vi "Actor Core.vi"(8 "error in":errorcluster, 11 "TestBench in":refnum<class "TestBench.lvclass">) -> (0 "error out":errorcluster, 3 "Actor out":refnum<class "Actor.lvclass">)   [LabVIEW 2019, in "TestBench.lvlib" / "TestBench.lvclass"]
doc: "(<B>Filename</B>: Actor Framework.lvlib:Actor.lvclass:Actor Core.vi)\n\nReceives messages to the actor, reacts to them, and initiates any error handling that may shut the actor down.\n\nDescendant classes may override this VI to append parallel tasks for the actor to complete while it handles messages. Overrides use the Call Parent Method node."
uses:
  TestBench.lvclass
  C:/Program Files (x86)/National Instruments/LabVIEW 2019/vi.lib/ActorFramework/Actor/Actor.lvclass
  <vilib>/ActorFramework/Actor/Actor.lvclass
  DataBase/DataBase/DataBase.lvclass
  EventRecorder/EventRecorder/EventRecorder.lvclass
  TestSetup/TestSetup/TestSetup.lvclass
  UserManagement/UserManagement/UserManagement.lvclass
  LocalReport/LocalReport/LocalReport.lvclass
  SignalProcessing/SignalProcessing/SignalProcessing.lvclass
  SoftwareSetup/SoftwareSetup/SoftwareSetup.lvclass
  SoftwareSetup/SoftwareSetup/DataBase.ctl
  SoftwareSetup/SoftwareSetup/Local Report.ctl
  SoftwareSetup/SoftwareSetup/Localization.ctl
  SoftwareSetup/SoftwareSetup/Preferences.ctl
  SoftwareSetup/SoftwareSetup/User Manager.ctl
  SoftwareSetup/SoftwareSetup/Multiple UUT Settings.ctl
  SoftwareSetup/SoftwareSetup/Sequence.ctl
  SystemSetup/SystemSetup/SystemSetup.lvclass
  Assert/Assert/Assert.lvclass
  TestRunner/TestRunner/TestRunner.lvclass
  TestBench.lvclass/TestBench.ctl
  HardwareSetup_model001/HardwareSetup_modle001/HardwareSetup_model001.lvclass
  D:/TestBench/SystemSetup/SystemSetup/SystemSetup.lvclass
  <vilib>/ActorFramework/Actor/Actor.lvclass/Actor.ctl
  <vilib>/ActorFramework/Message Enqueuer/Message Enqueuer.lvclass/Message Enqueuer.ctl
  UserManagement/UserManagement Messages/ActorCoreMassageEvent Msg/ActorCoreMassageEvent Msg.lvclass/ActorCoreMassageEvent Msg.ctl
  SystemSetup/SystemSetup Messages/ActorCoreEvent Msg/ActorCoreEvent Msg.lvclass/ActorCoreEvent Msg.ctl
  EventRecorder/EventRecorder Messages/ActorCoreEvent Msg/ActorCoreEvent Msg.lvclass/ActorCoreEvent Msg.ctl
  DataBase/DataBase Messages/ActorCoreEvent Msg/ActorCoreEvent Msg.lvclass/ActorCoreEvent Msg.ctl
  LocalReport/LocalReport Messages/InitializeReport Msg/InitializeReport Msg.lvclass/InitializeReport Msg.ctl
  DataBase/DataBase Messages/Initialize Msg/Initialize Msg.lvclass/Initialize Msg.ctl
  89e34157-fbcc-4783-a5bd-c972c4c63c1c.vi
  <vilib>/ActorFramework/Message Enqueuer/Init from Existing Queue.vi
  <vilib>/ActorFramework/Message Enqueuer/Enqueue.vi
  TestBench Messages/Stop Test Engine Actor Msg/Stop Test Engine Actor Msg.lvclass
  C:/Program Files (x86)/National Instruments/LabVIEW 2019/vi.lib/ActorFramework/Message/Message.lvclass
  <vilib>/ActorFramework/Stop Msg/Stop Msg.lvclass
  TestBench Messages/UI Initialize Msg/UI Initialize Msg.lvclass
  UserManagement/UserManagement Messages/Login Msg/Login Msg.lvclass
  TestBench Messages/Logout Msg/Logout Msg.lvclass
  UserManagement/UserManagement Messages/ActorCoreMassageEvent Msg/ActorCoreMassageEvent Msg.lvclass
  SystemSetup/SystemSetup Messages/ActorCoreEvent Msg/ActorCoreEvent Msg.lvclass
  EventRecorder/EventRecorder Messages/ActorCoreEvent Msg/ActorCoreEvent Msg.lvclass
  DataBase/DataBase Messages/ActorCoreEvent Msg/ActorCoreEvent Msg.lvclass
  TestBench Messages/Terminate Test Msg/Terminate Test Msg.lvclass
  TestBench Messages/SelectProductModle Msg/SelectProductModel Msg.lvclass
  TestBench Messages/ReadSerialNumber Msg/ReadSerialNumber Msg.lvclass
  LocalReport/LocalReport Messages/InitializeReport Msg/InitializeReport Msg.lvclass
  TestBench Messages/LunchTest Msg/LunchTest Msg.lvclass
  TestBench Messages/Change Sub Panel VI Msg/Change Sub Panel VI Msg.lvclass
  TestBench Messages/PopUp Msg/PopUp Msg.lvclass
  DataBase/DataBase Messages/Initialize Msg/Initialize Msg.lvclass
  <vilib>/ActorFramework/Message Priority Queue/Priority Enqueue.vi
  <vilib>/ActorFramework/Message Enqueuer/Message Enqueuer.lvclass
  SoftwareSetup/SoftwareSetup.lvlib
panel:
  in  "Socket List":i32(listbox)
  in  "Reconnection MySQL":bool
  in  "ShowScannerDialog":bool
  out "Slide":u32(slide)=17 scale=0.0..100.0
  out "CycleTime":dbl format="%.3f(s)"
  in  "Launch":bool
  in  "Break on Failure":enum32{"Yes", "No"}(radio)
  out "ProductType":string
  out "SequencePath":string
  out "Statistics":T1 {"Total" format="Total: %d"; "Yield" format="Yield: %.2f"; "Failed" format="Failed: %d"; "Pass" format="Pass: %d"}
  out "UserName":string
  out "StateBar":string
  # "SequencePath"
  # "ProductType"
  # "CycleTime"
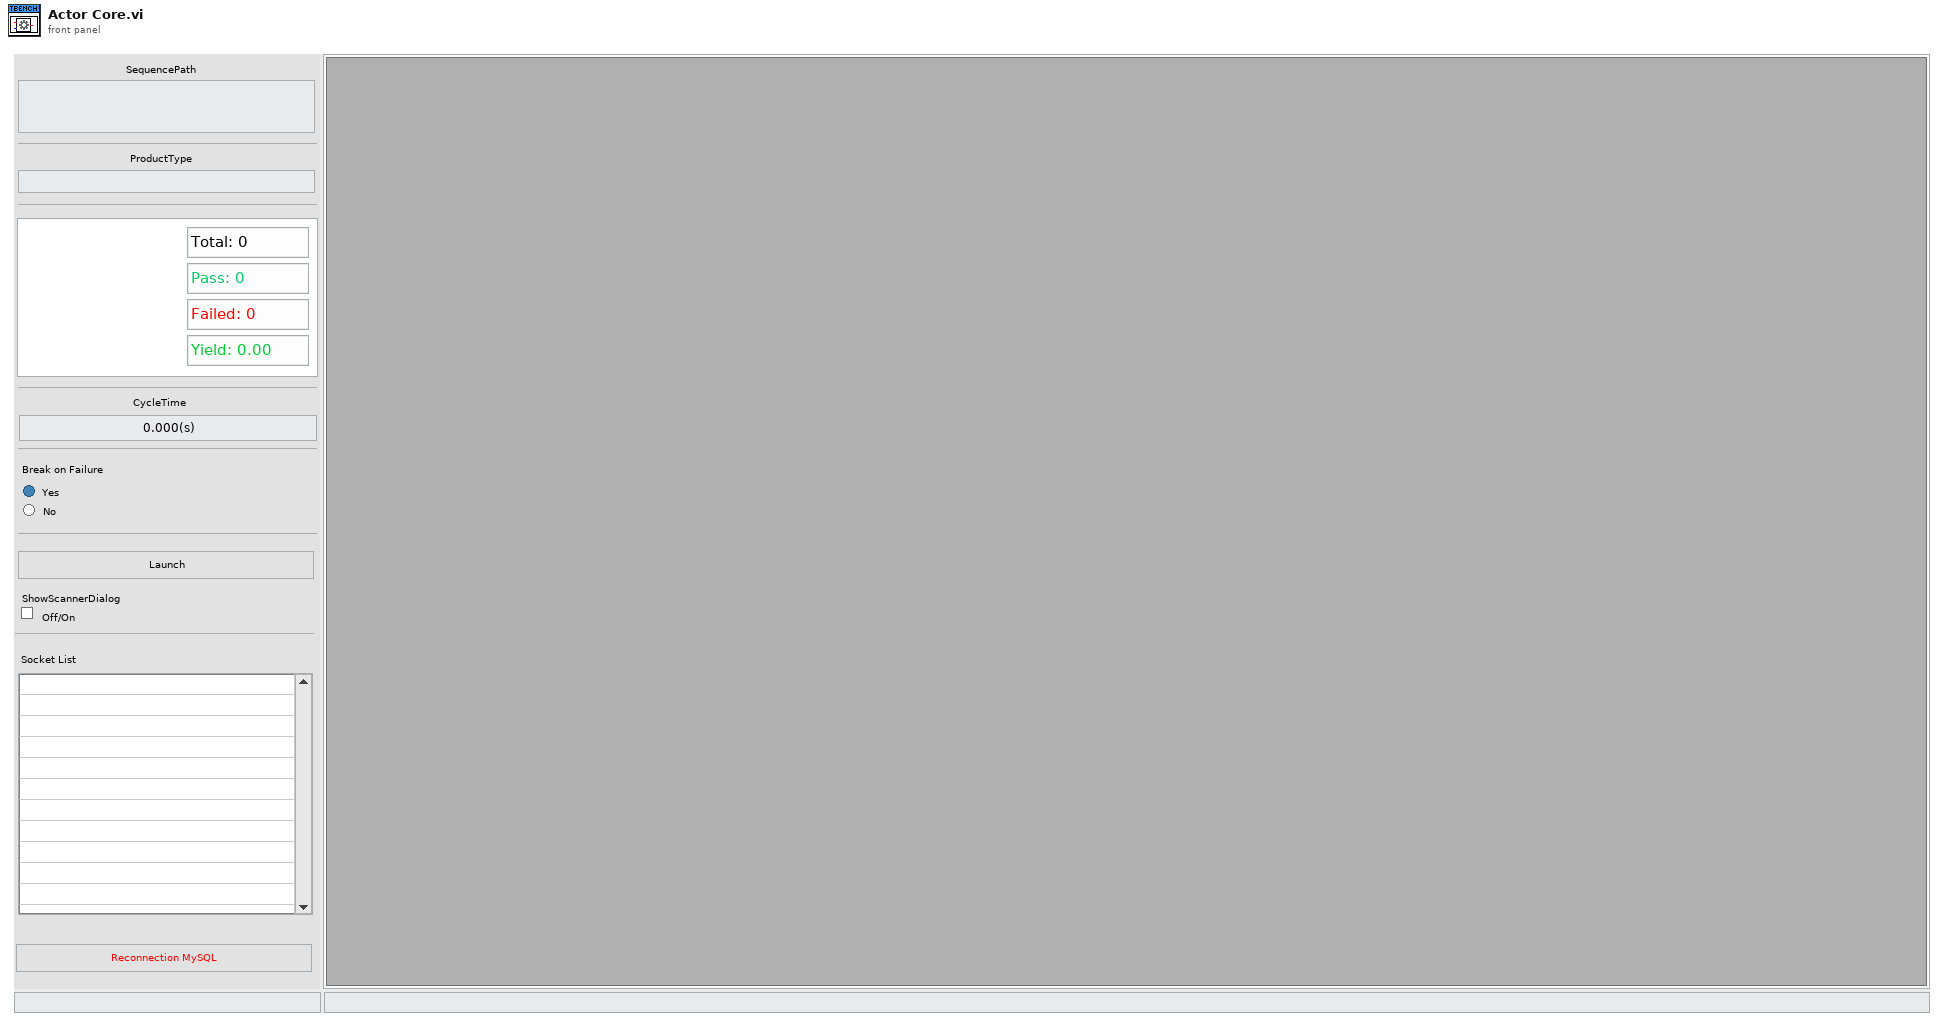
[diagram p1: front panel]
types:
  T1 = cluster{"2D Picture":picture, "Pass":u32, "Failed":u32, "Yield":dbl, "Total":u32}
  T2 = typedef "SoftwareSetup.lvlib/DataBase.ctl" = cluster{"Connection String Expression":string, "User ID":string, "Password":string}
  T3 = typedef "SoftwareSetup.lvlib/Local Report.ctl" = cluster{"Report Path":path, "Report  Format":enum16{"CSV", "XML", "PDF", "Excel", "TXT"}, "Disabled State":bool, "Customer name":string}
  T4 = typedef "SoftwareSetup.lvlib/Localization.ctl" = cluster{"Language":enum16{"English", "Chinese"}}
  T5 = typedef "SoftwareSetup.lvlib/Preferences.ctl" = cluster{"Station ID":string, "IP Address":string, "Password":string}
  T6 = typedef "SoftwareSetup.lvlib/User Manager.ctl" = cluster{"Current User Manager File":string, "Login on start":bool}
  T7 = typedef "SoftwareSetup.lvlib/Multiple UUT Settings.ctl" = cluster{"Number of Tests Sockets":u8, "Synchronization":enum16{"Don't Synchronize", "Serial", "Parallel", "One Thread Only"}}
  T8 = typedef "SoftwareSetup.lvlib/Sequence.ctl" = cluster{"Sequence Folder Path":path}
  T9 = cluster{"DataBase":T2, "Local Report":T3, "Localization":T4, "Preferences":T5, "User Manager":T6, "Multiple UUT Settings":T7, "Sequence":T8}
  T10 = enum32{"Invalid", "Standard", "Closed", "Hidden", "Minimized", "Maximized"}
  T11 = enum32{"invalid app kind", "Development System", "Run Time System", "Student Edition", "Embedded LabVIEW", "Evaluation", "Custom"}
  T12 = cluster{"User ID":string, "ConnectString":string, "Password":string}
  T13 = cluster{"Core":cluster{"Current VI Reference":refnum<vi>, "Close Panel on Exit?":bool}, "DataBase":T2, "Local Report":T3, "Localization":T4, "Preferences":T5, "User Manager":T6}
  T14 = cluster{"Current VI Reference":refnum<vi>, "Close Panel on Exit?":bool}
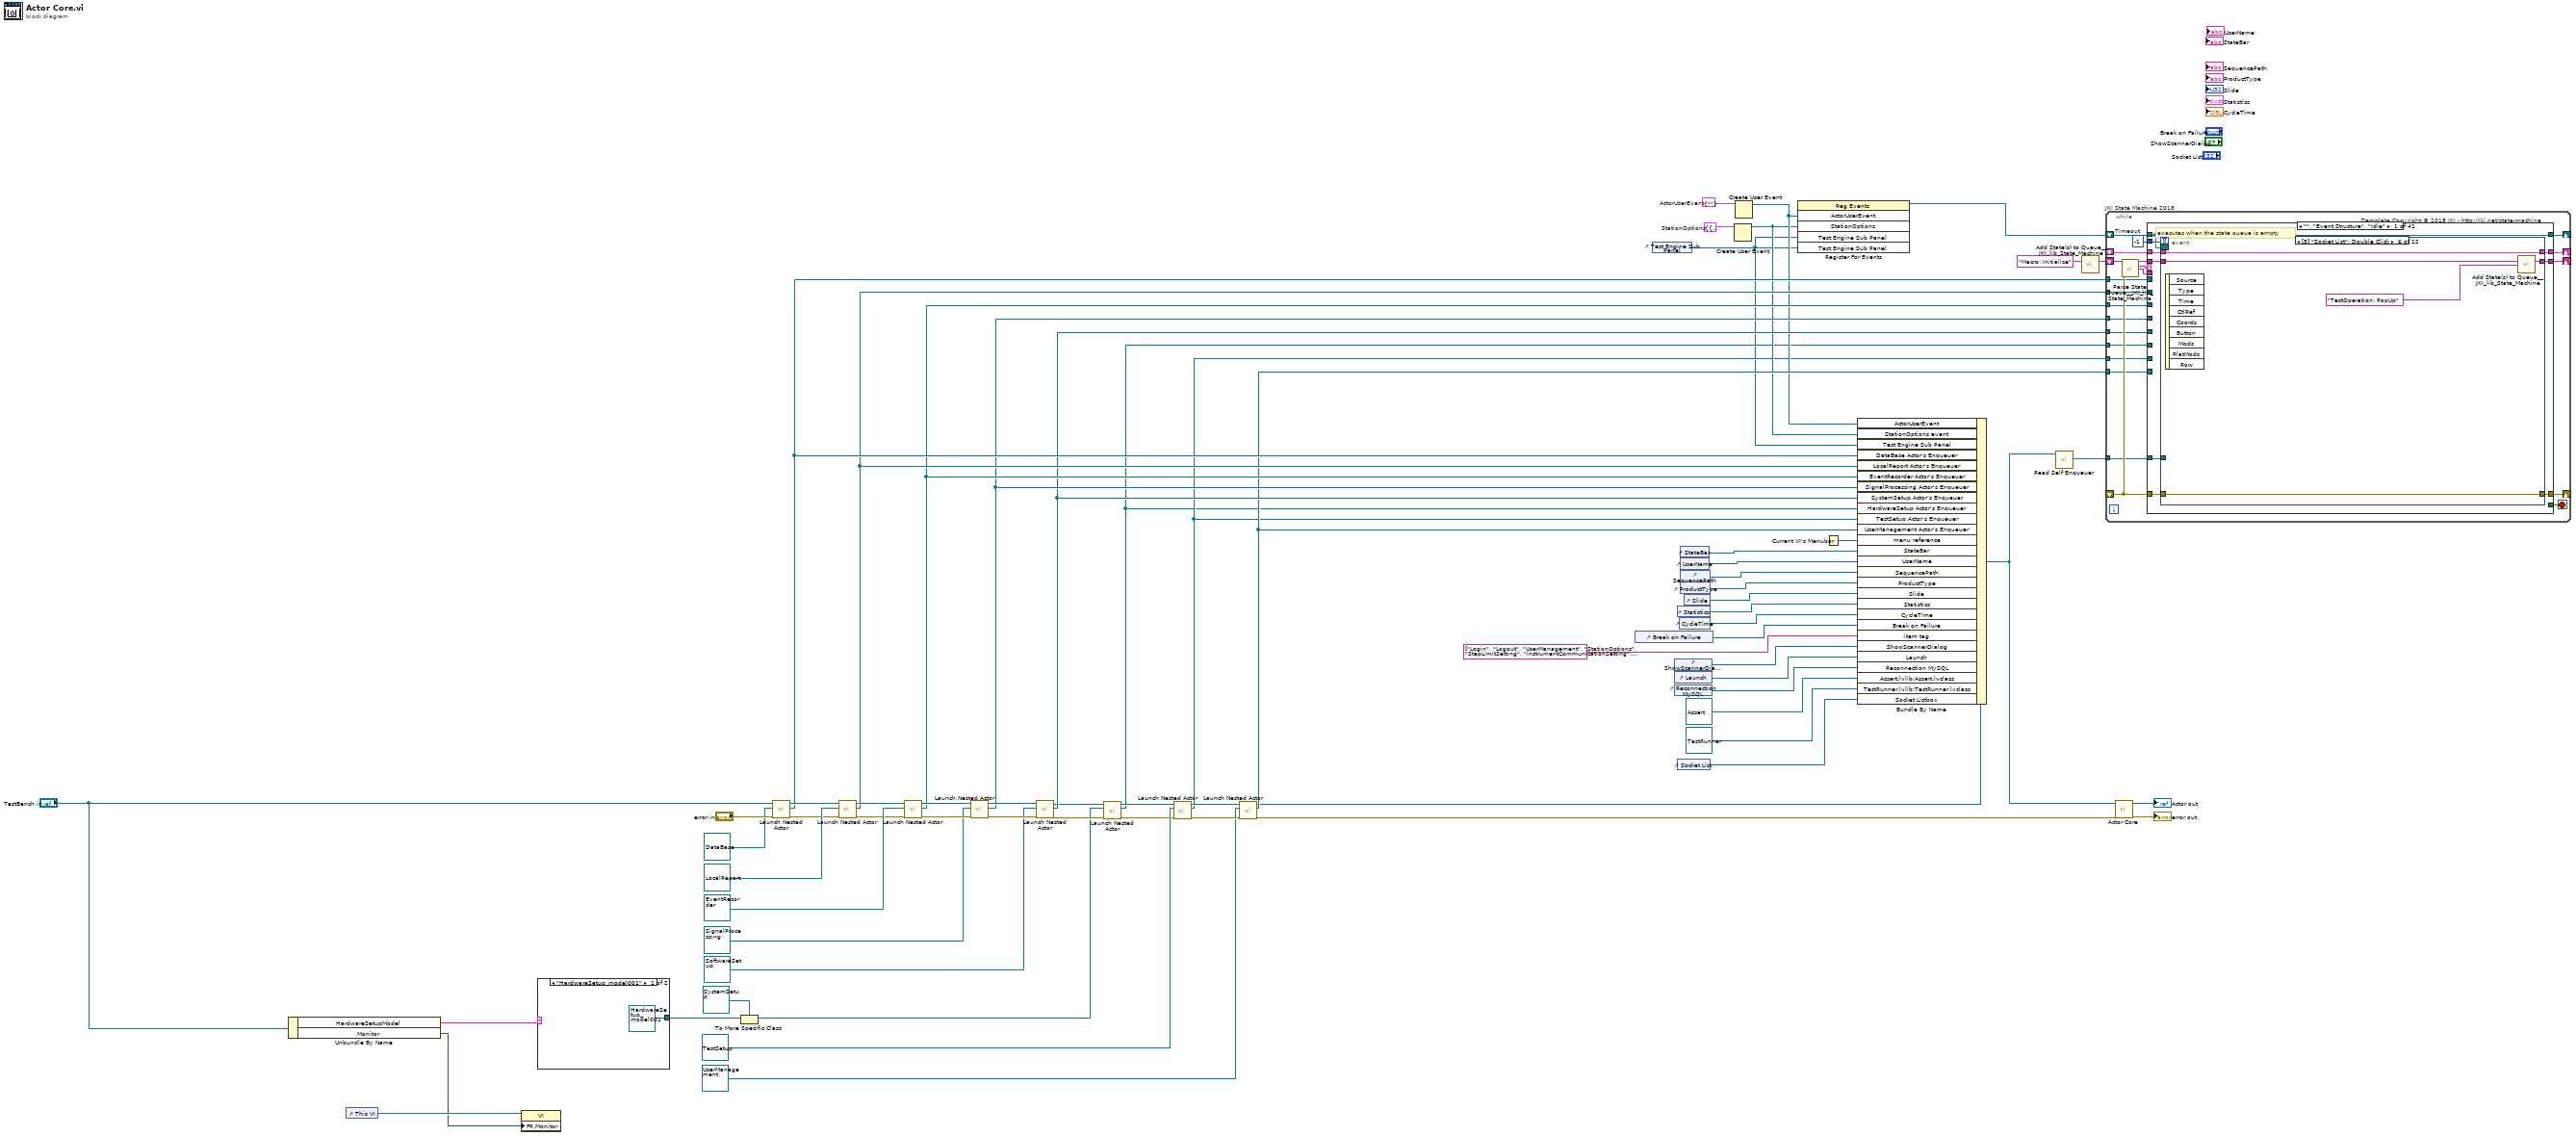
[diagram p0: block diagram]
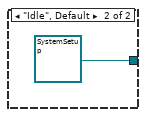
[diagram p2: hidden frame]
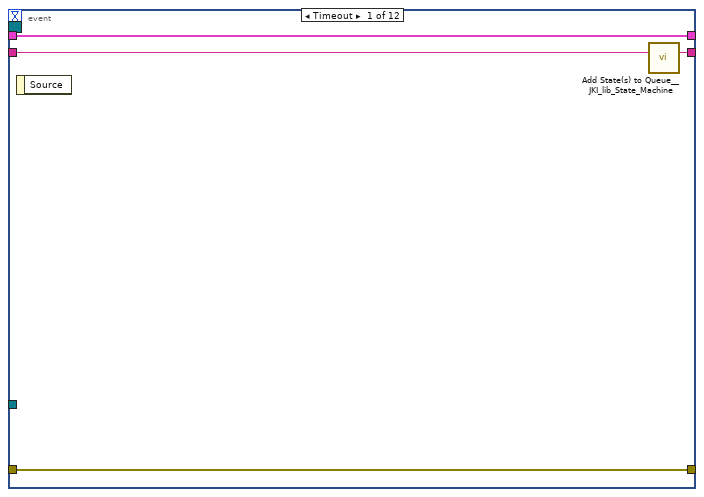
[diagram p3: hidden frame]
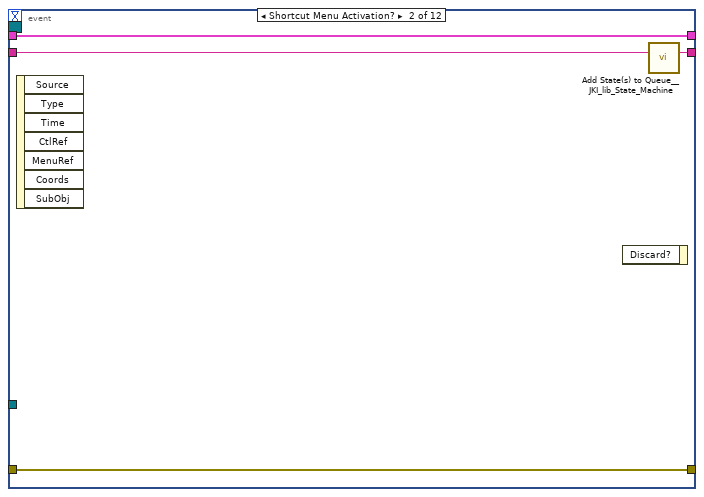
[diagram p4: hidden frame]
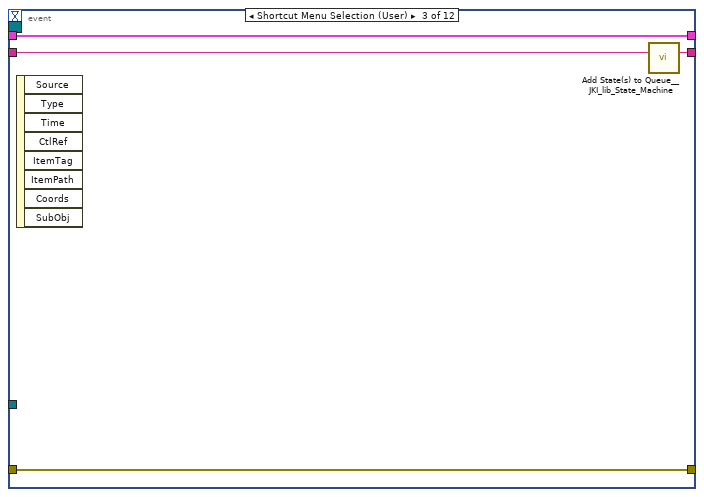
[diagram p5: hidden frame]
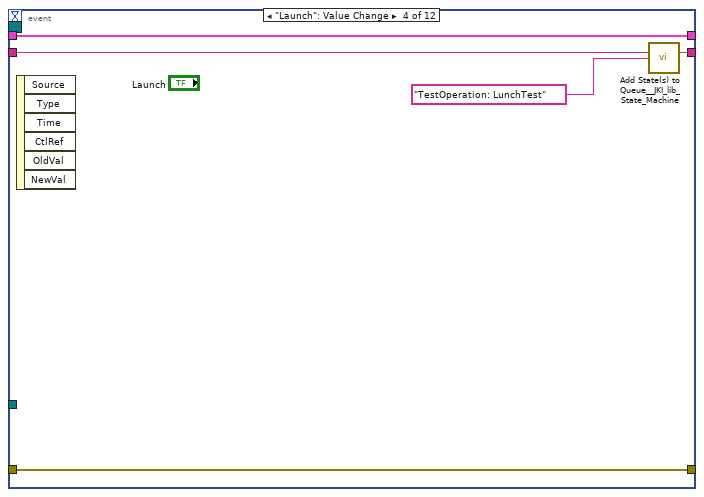
[diagram p6: hidden frame]
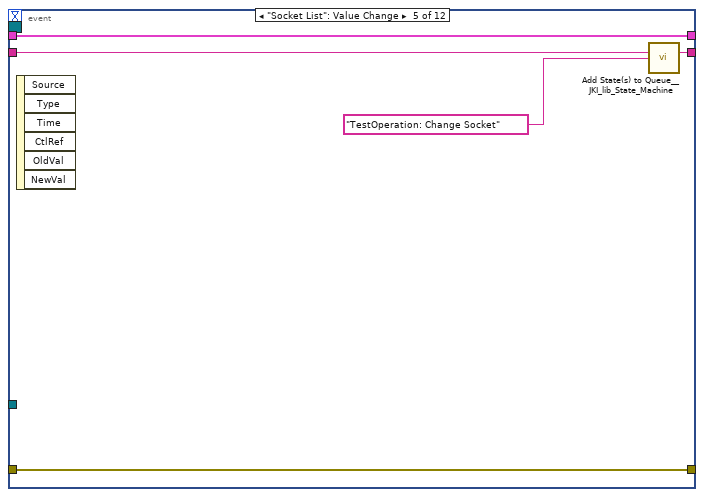
[diagram p7: hidden frame]
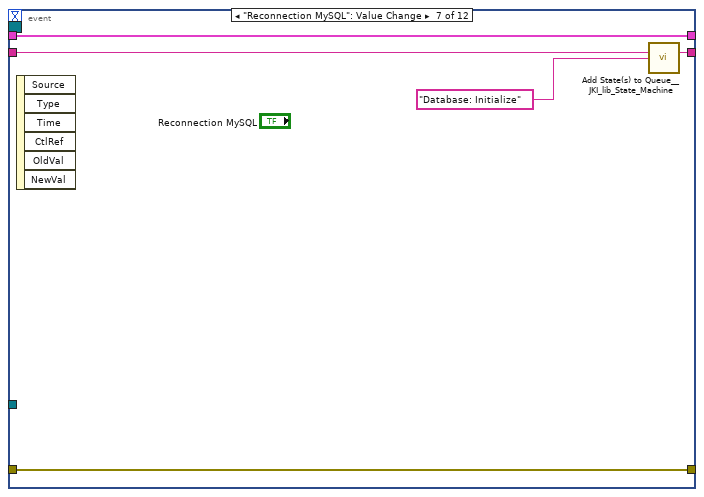
[diagram p8: hidden frame]
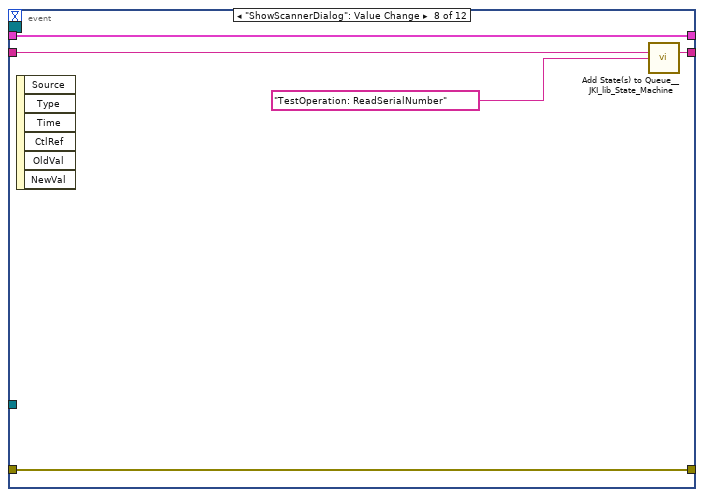
[diagram p9: hidden frame]
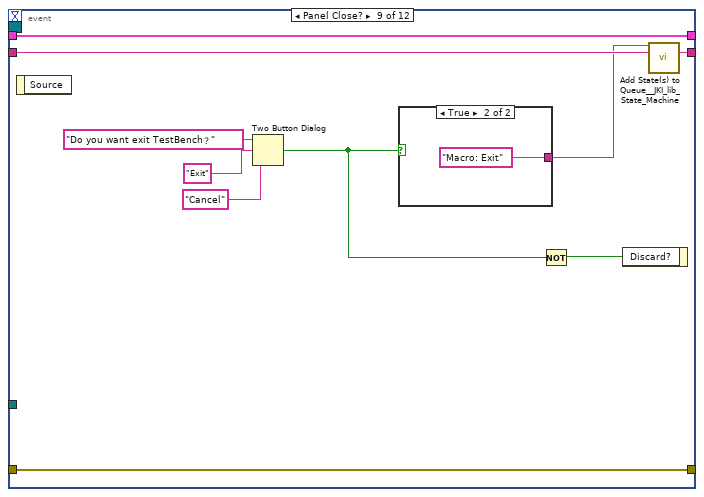
[diagram p10: hidden frame]
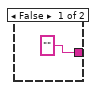
[diagram p11: hidden frame]
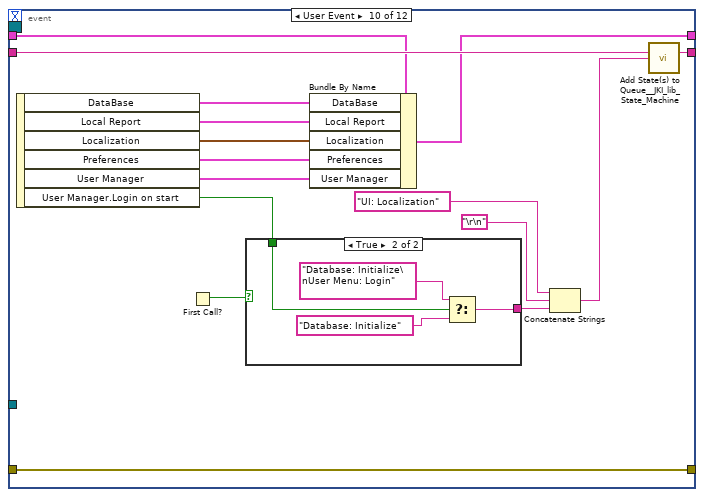
[diagram p12: hidden frame]
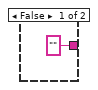
[diagram p13: hidden frame]
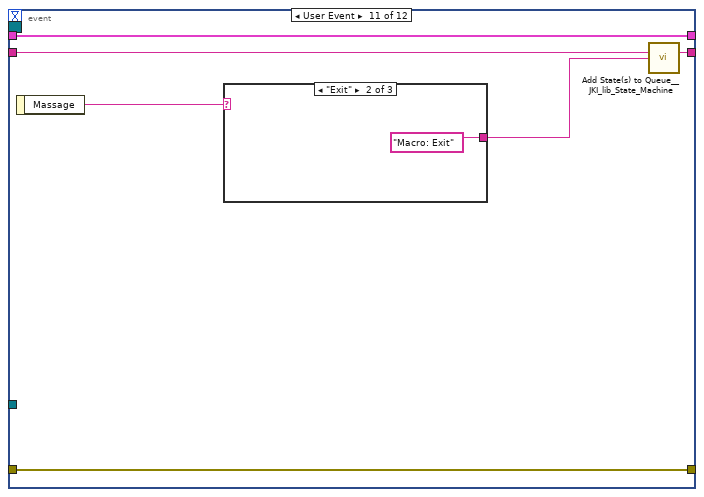
[diagram p14: hidden frame]
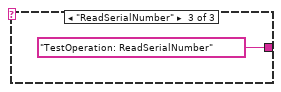
[diagram p16: hidden frame]
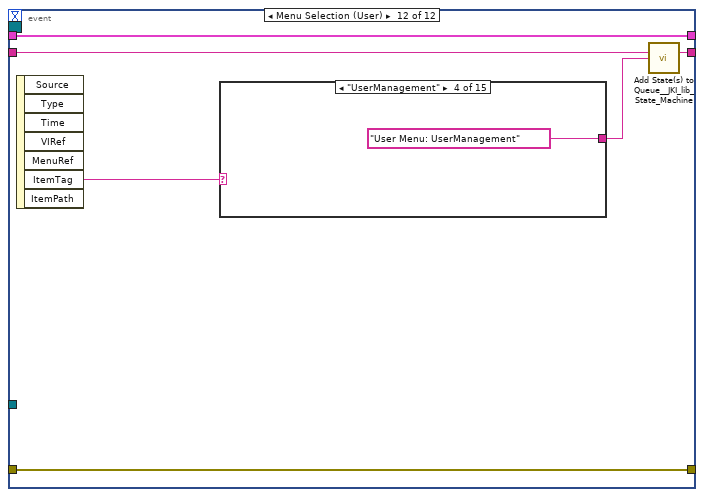
[diagram p17: hidden frame]
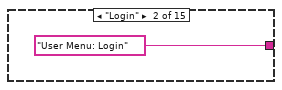
[diagram p19: hidden frame]
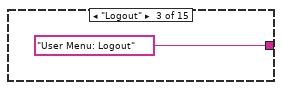
[diagram p20: hidden frame]
diagram:
  w27 = T9 {"DataBase"={"Connection String Expression"="", "User ID"="", "Password"=""}, "Local Report"={"Report Path"=path "", "Report  Format"=enum."CSV", "Disabled State"=FALSE, "Customer name"=""}, "Localization"={"Language"=enum."English"}, "Preferences"={"Station ID"="", "IP Address"="", "Password"=""}, "User Manager"={"Current User Manager File"="", "Login on start"=FALSE}, "Multiple UUT Settings"={"Number of Tests Sockets"=1, "Synchronization"=enum."Serial"}, "Sequence"={"Sequence Folder Path"=path ""}}  # StationOptions
  w55 = cluster{"Massage":string} {"Massage"=""}  # ActorUserEvent
  n1 = Unbundle By Name("TestBench in") -> ("HardwareSetupModel"=w10:string, "Monitor"=w8:u16)
  n2 = control-ref of="This VI"() -> (w9:refnum<vi>)
  n3 = property class="VI"(reference=w9, "FP.Monitor"=w8) -> ()  [unwired: 1 in, 2 out]
  n4 = case shown="\"HardwareSetup_model001\"" w10 {
    tunnel: [refnum<class "HardwareSetup_model001.lvclass"> refnum ("HardwareSetup_model001.lvlib:HardwareSetup_model001.lvclass") refnum<class "SystemSetup.lvclass"> refnum ("SystemSetup.lvlib:SystemSetup.lvclass")] -> w11
    frame "HardwareSetup_model001" {
    }
    frame "Idle", Default {
    }
  }
  n5 = To More Specific Class(target class=refnum<class "SystemSetup.lvclass"> refnum ("SystemSetup.lvlib:SystemSetup.lvclass"), reference=w11) -> (specific class reference=w12:refnum<class "SystemSetup.lvclass">)  [unwired: 1 in, 1 out]
  n6 = call <vilib>:"Launch Nested Actor.vi"("error in (no error)"="error in", "Nested Actor"=refnum<class "DataBase.lvclass"> refnum ("DataBase.lvlib:DataBase.lvclass"), "Caller Actor in"="TestBench in") -> ("error out"=w42:errorcluster, "Nested Actor's Enqueuer"=w35:refnum<class "Message Enqueuer.lvclass">, "Caller Actor out"=w44:refnum<class "TestBench.lvclass">)  [unwired: 6 in]
  n7 = call <vilib>:"Launch Nested Actor.vi"("error in (no error)"=w42, "Nested Actor"=refnum<class "LocalReport.lvclass"> refnum ("LocalReport.lvlib:LocalReport.lvclass"), "Caller Actor in"=w44) -> ("error out"=w40:errorcluster, "Nested Actor's Enqueuer"=w34:refnum<class "Message Enqueuer.lvclass">, "Caller Actor out"=w41:refnum<class "TestBench.lvclass">)  [unwired: 6 in]
  n8 = call <vilib>:"Launch Nested Actor.vi"("error in (no error)"=w40, "Nested Actor"=refnum<class "EventRecorder.lvclass"> refnum ("EventRecorder.lvlib:EventRecorder.lvclass"), "Caller Actor in"=w41) -> ("error out"=w37:errorcluster, "Nested Actor's Enqueuer"=w33:refnum<class "Message Enqueuer.lvclass">, "Caller Actor out"=w39:refnum<class "TestBench.lvclass">)  [unwired: 6 in]
  n9 = call <vilib>:"Launch Nested Actor.vi"("error in (no error)"=w37, "Nested Actor"=refnum<class "SignalProcessing.lvclass"> refnum ("SignalProcessing.lvlib:SignalProcessing.lvclass"), "Caller Actor in"=w39) -> ("error out"=w36:errorcluster, "Nested Actor's Enqueuer"=w32:refnum<class "Message Enqueuer.lvclass">, "Caller Actor out"=w38:refnum<class "TestBench.lvclass">)  [unwired: 6 in]
  n10 = call <vilib>:"Launch Nested Actor.vi"("error in (no error)"=w36, "Nested Actor"=refnum<class "SoftwareSetup.lvclass"> refnum ("SoftwareSetup.lvlib:SoftwareSetup.lvclass"), "Caller Actor in"=w38) -> ("error out"=w22:errorcluster, "Nested Actor's Enqueuer"=w31:refnum<class "Message Enqueuer.lvclass">, "Caller Actor out"=w23:refnum<class "TestBench.lvclass">)  [unwired: 6 in]
  n11 = call <vilib>:"Launch Nested Actor.vi"("error in (no error)"=w22, "Nested Actor"=w12, "Caller Actor in"=w23) -> ("error out"=w20:errorcluster, "Nested Actor's Enqueuer"=w18:refnum<class "Message Enqueuer.lvclass">, "Caller Actor out"=w21:refnum<class "TestBench.lvclass">)  [unwired: 6 in]
  n12 = call <vilib>:"Launch Nested Actor.vi"("error in (no error)"=w20, "Nested Actor"=refnum<class "TestSetup.lvclass"> refnum ("TestSetup.lvlib:TestSetup.lvclass"), "Caller Actor in"=w21) -> ("error out"=w59:errorcluster, "Nested Actor's Enqueuer"=w19:refnum<class "Message Enqueuer.lvclass">, "Caller Actor out"=w60:refnum<class "TestBench.lvclass">)  [unwired: 6 in]
  n13 = call <vilib>:"Launch Nested Actor.vi"("error in (no error)"=w59, "Nested Actor"=refnum<class "UserManagement.lvclass"> refnum ("UserManagement.lvlib:UserManagement.lvclass"), "Caller Actor in"=w60) -> ("error out"=w6:errorcluster, "Nested Actor's Enqueuer"=w30:refnum<class "Message Enqueuer.lvclass">, "Caller Actor out"=w7:refnum<class "TestBench.lvclass">)  [unwired: 6 in]
  n14 = control-ref of="Break on Failure"() -> (w46:refnum<vi>)
  n15 = control-ref of="Test Engine Sub Panel"() -> (w4:refnum<vi>)
  n16 = control-ref of="Launch"() -> (w15:refnum<vi>)
  n17 = control-ref of="Reconnection MySQL"() -> (w14:refnum<vi>)
  n18 = control-ref of="ShowScannerDialog"() -> (w16:refnum<vi>)
  n19 = control-ref of="Statistics"() -> (w48:refnum<vi>)
  n20 = control-ref of="Socket List"() -> (w1:refnum<vi>)
  n21 = control-ref of="CycleTime"() -> (w47:refnum<vi>)
  n22 = control-ref of="StateBar"() -> (w53:refnum<vi>)
  n23 = control-ref of="UserName"() -> (w52:refnum<vi>)
  n24 = control-ref of="SequencePath"() -> (w51:refnum<vi>)
  n25 = control-ref of="ProductType"() -> (w50:refnum<vi>)
  n26 = control-ref of="Slide"() -> (w49:refnum<vi>)
  n27 = Create User Event(user event datatype=w27) -> (user event=w25:refnum<user-event>)  [unwired: 1 in, 1 out]
  n28 = Create User Event(user event datatype=w55) -> (user event=w26:refnum<user-event>)  [unwired: 1 in, 1 out]
  n29 = register-events(w26, w25, w4, w4) -> (reference out=w54:refnum<event-registration>)  [unwired: 2 in, 1 out]
  n30 = Current VI's Menubar() -> (w5:refnum<k9>)
  n31 = Bundle By Name(cluster=w7, "ActorUserEvent"=w26, "StationOptions event"=w25, "Test Engine Sub Panel"=w4, "DataBase Actor's Enqueuer"=w35, "LocalReport Actor's Enqueuer"=w34, "EventRecorder Actor's Enqueuer"=w33, "SignalProcessing Actor's Enqueuer"=w32, "SystemSetup Actor's Enqueuer"=w31, "HardwareSetup Actor's Enqueuer"=w18, "TestSetup Actor's Enqueuer"=w19, "UserManagement Actor's Enqueuer"=w30, "menu reference"=w5, "StateBar"=w53, "UserName"=w52, "SequencePath"=w51, "ProductType"=w50, "Slide"=w49, "Statistics"=w48, "CycleTime"=w47, "Break on Failure"=w46, "item tag"=string[] ["Login", "Logout", "UserManagement", "StationOptions", "StepLimitSetting", "InstrumentCommunicationSetting", "LunchTest", "Terminate", "DebugUI", "TestParameterEdit"], "ShowScannerDialog"=w16, "Launch"=w15, "Reconnection MySQL"=w14, "Assert.lvlib:Assert.lvclass"=refnum<class "Assert.lvclass"> refnum, "TestRunner.lvlib:TestRunner.lvclass"=refnum<class "TestRunner.lvclass"> refnum, "Socket Listbox"=w1) -> (w62:refnum<class "TestBench.lvclass">)
  n32 = call <vilib>:"Read Self Enqueuer.vi"("Actor"=w62) -> ("Self Enqueuer"=w63:refnum<class "Message Enqueuer.lvclass">)  [unwired: 10 in]
  n33 = call <vilib>:"Add State(s) to Queue__JKI_lib_State_Machine.vi"("State(s) in (\"\")"="Macro: Initialize") -> ("States Out"=w65:string)  [unwired: 14 in]
  n34 = while "JKI State Machine 2018" {
    shift-right: [w84] -> _
    shift-left: _ -> [w83]
    shift-right: [w87] -> _
    shift-left: _ -> [w81]
    shift-right: [w86] -> _
    shift-left: w65 -> [w88]
    tunnel: w63 -> [w80]
    tunnel: w35 -> [w79]
    tunnel: w33 -> [w78]
    tunnel: w31 -> [w77]
    tunnel: w19 -> [w76]
    tunnel: w30 -> [w75]
    shift-right: [w74] -> _
    shift-left: w54 -> [w73]
    tunnel: w34 -> [w72]
    tunnel: w32 -> [w71]
    tunnel: w18 -> [w70]
    stop <- w85 stop-if-true
    w82 = -1  # Timeout
    # "Template Copyright © 2018 JKI - http://jki.net/state-machine"
    n35 = call <vilib>:"Parse State Queue__JKI_lib_State_Machine.vi"("State Queue"=w88, "Error In (no error)"=w81) -> ("Remaining States"=w90:string, "Current State"=w91:string, "Arguments"=w89:string)  [unwired: 11 in]
    n36 = case shown="\"\", \"Event Structure\", \"Idle\"" w91 {
      selector: w91 -> [_ _ w205 _ _ _ _ _ _ _ _ _ _ _ _ _ _ _ _ _ _ _ _ _ _ _ _ _ _ _ _ _ _ _ _ _ _ _ _ _ _]
      tunnel: w90 -> [w100 w203 w209 w229 w236 w253 w259 w270 w277 w282 w298 w314 w319 w325 w332 w341 w349 w419 w425 w436 w441 w447 w453 w460 w467 w474 w481 w488 w495 w501 w507 w521 w541 w552 w558 w564 w576 w583 w590 w595 w606]
      tunnel: w89 -> [_ _ _ _ _ _ _ _ _ _ _ _ _ _ w327 _ w345 _ _ _ _ _ _ _ _ _ _ _ _ _ _ _ _ _ _ _ _ _ _ _ _]
      tunnel: w83 -> [w98 w200 w207 w222 w233 w251 w256 _ w272 w279 w296 w312 w316 w320 w330 w338 w346 w416 w422 w433 w438 w442 w450 w457 w464 w471 w478 w485 w492 w498 w504 w519 w539 w549 w555 w561 w571 w580 w587 w592 w602]
      tunnel: [w97 w201 w211 w226 errorcluster {"status"=FALSE, "code"=0, "source"=""} ("error out") w250 w257 w267 w273 w280 w290 w309 w317 w323 w328 w337 w342 w417 w423 w434 w439 w445 w451 w458 w465 w472 w479 w486 w493 w499 w505 w511 w528 w550 w556 w562 w567 w577 w584 w591 w596] -> w87
      tunnel: w81 -> [w96 w201 w210 w226 w232 w250 w257 w267 w274 w280 w291 w310 w317 w323 w329 w337 w347 w417 w423 w434 w439 w445 w451 w458 w465 w472 w479 w486 w493 w499 w505 w517 w529 w550 w556 w562 w568 w578 w585 w591 w596]
      tunnel: [w99 w202 w208 w228 w235 w252 w258 w269 w276 w281 w297 w313 w318 w324 w331 w340 w348 w418 w424 w435 w440 w446 w452 w459 w466 w473 w480 w487 w494 w500 w506 w520 w540 w551 w557 w563 w575 w582 w589 w594 w605] -> w86
      tunnel: [_ _ _ _ _ TRUE _ _ _ _ _ _ _ _ _ _ _ _ _ _ _ _ _ _ _ _ _ _ _ _ _ _ _ _ _ _ _ _ _ _ _] -> w85
      tunnel: [w95 w200 w207 w227 w233 w251 w256 w268 w272 w279 w296 w312 w316 w320 w330 w338 w346 w416 w422 w433 w438 w442 w450 w457 w464 w471 w478 w485 w492 w498 w504 w519 w539 w549 w555 w561 w571 w580 w587 w592 w602] -> w84
      tunnel: w82 -> [w94 _ _ _ _ _ _ _ _ _ _ _ _ _ _ _ _ _ _ _ _ _ _ _ _ _ _ _ _ _ _ _ _ _ _ _ _ _ _ _ _]
      tunnel: w80 -> [w92 _ _ _ _ w238 _ _ _ _ w292 w299 _ w321 _ _ _ _ _ _ _ _ w448 _ _ _ _ _ _ _ w502 _ _ _ w553 w559 w573 w579 w586 _ _]
      tunnel: w79 -> [_ _ _ _ _ w247 _ _ _ _ w294 w308 _ _ _ _ _ _ _ _ _ _ _ _ _ _ _ _ w490 _ _ _ _ _ _ _ _ _ _ _ w603]
      tunnel: w78 -> [_ _ _ _ _ w245 _ _ _ _ w288 w306 _ _ _ _ _ _ _ _ _ _ _ _ _ _ _ w483 _ _ _ _ _ _ _ _ _ _ _ _ _]
      tunnel: w77 -> [_ _ _ _ _ w243 _ _ _ _ w286 w304 _ _ _ _ _ _ _ _ _ _ _ _ w462 _ _ _ _ _ _ _ _ _ _ _ _ _ _ _ _]
      tunnel: w76 -> [_ _ _ _ _ w241 _ _ _ _ w284 w302 _ _ _ _ _ _ _ _ _ _ _ _ _ w468 _ _ _ _ _ _ _ _ _ _ _ _ _ _ _]
      tunnel: w75 -> [_ _ _ _ _ w240 _ _ _ _ w283 w301 _ _ _ _ _ _ _ _ _ w443 _ w455 _ _ _ _ _ _ _ _ _ _ _ _ _ _ _ _ _]
      tunnel: [w93 w199 w204 w216 w230 w248 w255 w265 w271 w278 w295 w311 w315 w322 w326 w339 w344 w415 w420 w426 w437 w444 w449 w456 w463 w470 w477 w484 w491 w497 w503 w518 w538 w548 w554 w560 w574 w581 w588 w593 w604] -> w74
      tunnel: w73 -> [w93 w199 w204 w216 w230 w248 w255 w265 w271 w278 w295 w311 w315 w322 w326 w339 w344 w415 w420 w426 w437 w444 w449 w456 w463 w470 w477 w484 w491 w497 w503 w518 w538 w548 w554 w560 w574 w581 w588 w593 w604]
      tunnel: w72 -> [_ _ _ _ _ w246 _ _ _ _ w289 w307 _ _ _ _ _ _ _ _ _ _ _ _ _ _ _ _ _ _ _ _ _ _ _ _ w572 _ _ _ _]
      tunnel: w71 -> [_ _ _ _ _ w244 _ _ _ _ w287 w305 _ _ _ _ _ _ _ _ _ _ _ _ _ _ _ _ _ _ _ _ _ _ _ _ _ _ _ _ _]
      tunnel: w70 -> [_ _ _ _ _ w242 _ _ _ _ w285 w303 _ _ _ _ _ _ _ _ _ _ _ _ _ _ w475 _ _ _ _ _ _ _ _ _ _ _ _ _ _]
      frame "", "Event Structure", "Idle" {
        # "executes when the state queue is empty"
        n37 = event shown="[5] \"Socket List\": Double Click" {
          selector: w93 -> [_ _ _ _ _ _ _ _ _ _ _ _]
          dyn-events: _ -> [_ _ _ _ _ _ _ _ _ _ _ _]
          timeout: w94 -> [_ _ _ _ _ _ _ _ _ _ _ _]
          tunnel: w100 -> [w104 w108 w112 w117 w122 w127 w132 w137 w147 w165 w176 w184]
          tunnel: [w103 w107 w111 w116 w121 w126 w131 w136 w146 w164 w175 w183] -> w99
          tunnel: w98 -> [w101 w105 w109 w114 w119 w124 w129 w134 w144 w162 w173 w181]
          tunnel: [w102 w106 w110 w115 w120 w125 w130 w135 w145 w163 w174 w182] -> w97
          tunnel: w96 -> [w102 w106 w110 w115 w120 w125 w130 w135 w145 w163 w174 w182]
          tunnel: [w101 w105 w109 w114 w119 w124 w129 w134 w144 w156 w173 w181] -> w95
          tunnel: w92 -> [_ _ _ _ _ _ _ _ _ _ _ _]
          event Timeout {
            n38 = event-data() -> ()  [unwired: 1 in, 1 out]
            n39 = call <vilib>:"Add State(s) to Queue__JKI_lib_State_Machine.vi"("State(s) in (\"\")"=w104) -> ("States Out"=w103:string)  [unwired: 14 in]
          }
          event Shortcut Menu Activation? {
            n40 = event-data() -> ()  [unwired: 1 in, 7 out]
            n41 = event-data() -> ()  [unwired: 2 in, 1 out]
            n42 = call <vilib>:"Add State(s) to Queue__JKI_lib_State_Machine.vi"("State(s) in (\"\")"=w108) -> ("States Out"=w107:string)  [unwired: 14 in]
          }
          event Shortcut Menu Selection (User) {
            n43 = event-data() -> ()  [unwired: 1 in, 8 out]
            n44 = call <vilib>:"Add State(s) to Queue__JKI_lib_State_Machine.vi"("State(s) in (\"\")"=w112) -> ("States Out"=w111:string)  [unwired: 14 in]
          }
          event "Launch": Value Change {
            n45 = event-data() -> ()  [unwired: 1 in, 6 out]
            n46 = call <vilib>:"Add State(s) to Queue__JKI_lib_State_Machine.vi"("State(s) in (\"\")"=w117, "State(s) at Back (\"\")"="TestOperation: LunchTest" ("State(s) at Back (\"\")")) -> ("States Out"=w116:string)  [unwired: 13 in]
          }
          event "Socket List": Value Change {
            n47 = event-data() -> ()  [unwired: 1 in, 6 out]
            n48 = call <vilib>:"Add State(s) to Queue__JKI_lib_State_Machine.vi"("State(s) in (\"\")"=w122, "State(s) at Back (\"\")"="TestOperation: Change Socket" ("State(s) at Back (\"\")")) -> ("States Out"=w121:string)  [unwired: 13 in]
          }
          event "Socket List": Double Click {
            n49 = event-data() -> ()  [unwired: 1 in, 9 out]
            n50 = call <vilib>:"Add State(s) to Queue__JKI_lib_State_Machine.vi"("State(s) in (\"\")"=w127, "State(s) at Back (\"\")"="TestOperation: PopUp" ("State(s) at Back (\"\")")) -> ("States Out"=w126:string)  [unwired: 13 in]
          }
          event "Reconnection MySQL": Value Change {
            n51 = event-data() -> ()  [unwired: 1 in, 6 out]
            n52 = call <vilib>:"Add State(s) to Queue__JKI_lib_State_Machine.vi"("State(s) in (\"\")"=w132, "State(s) at Back (\"\")"="Database: Initialize" ("State(s) at Back (\"\")")) -> ("States Out"=w131:string)  [unwired: 13 in]
          }
          event "ShowScannerDialog": Value Change {
            n53 = event-data() -> ()  [unwired: 1 in, 6 out]
            n54 = call <vilib>:"Add State(s) to Queue__JKI_lib_State_Machine.vi"("State(s) in (\"\")"=w137, "State(s) at Back (\"\")"="TestOperation: ReadSerialNumber" ("State(s) at Back (\"\")")) -> ("States Out"=w136:string)  [unwired: 13 in]
          }
          event Panel Close? {
            n55 = event-data() -> ()  [unwired: 1 in, 1 out]
            n56 = Two Button Dialog(message="Do you want exit TestBench？", 1:"Cancel" ("F button name (\"Cancel\")"), 2:"Exit" ("T button name (\"OK\")")) -> (T button?=w141:bool)
            n57 = case shown="True" w141 {
              tunnel: ["" "Macro: Exit"] -> w138
              frame False {
              }
              frame True {
              }
            }
            n58 = Not(x=w141) -> (.not. x?=w139:bool)
            n59 = event-data("Discard?"=w139) -> ()  [unwired: 1 in, 1 out]
            n60 = call <vilib>:"Add State(s) to Queue__JKI_lib_State_Machine.vi"("State(s) in Front (\"\")"=w138, "State(s) in (\"\")"=w147) -> ("States Out"=w146:string)  [unwired: 13 in]
          }
          event User Event {
            n61 = event-data() -> ("DataBase"=w161:T2, "Local Report"=w160:T3, "Localization"=w159:T4, "Preferences"=w158:T5, "User Manager"=w157:T6, "User Manager.Login on start"=w155:bool)  [unwired: 1 in]
            n62 = First Call?() -> (First Call?: T/F=w154:bool)
            n63 = case shown="True" w154 {
              tunnel: w155 -> [_ w170]
              tunnel: ["" w168] -> w153
              frame False {
              }
              frame True {
                n64 = Select(t="Database: Initialize\nUser Menu: Login", s=w170, f="Database: Initialize") -> (s? t:f=w168:string)
              }
            }
            n65 = Bundle By Name(cluster=w162, "DataBase"=w161, "Local Report"=w160, "Localization"=w159, "Preferences"=w158, "User Manager"=w157) -> (w156:T13)
            n66 = Concatenate Strings("UI: Localization" ("string"), "\r\n", w153) -> (w152:string)
            n67 = call <vilib>:"Add State(s) to Queue__JKI_lib_State_Machine.vi"("State(s) in (\"\")"=w165, "State(s) at Back (\"\")"=w152) -> ("States Out"=w164:string)  [unwired: 13 in]
          }
          event User Event {
            n68 = event-data() -> ("Massage"=w172:string)  [unwired: 1 in]
            n69 = case shown="\"Exit\"" w172 {
              tunnel: [_ "Macro: Exit" "TestOperation: ReadSerialNumber"] -> w171
              frame "Idle", Default {
              }
              frame "Exit" {
              }
              frame "ReadSerialNumber" {
              }
            }
            n70 = call <vilib>:"Add State(s) to Queue__JKI_lib_State_Machine.vi"("State(s) in (\"\")"=w176, "State(s) at Back (\"\")"=w171) -> ("States Out"=w175:string)  [unwired: 13 in]
          }
          event Menu Selection (User) {
            n71 = event-data() -> ("ItemTag"=w179:string)  [unwired: 1 in, 6 out]
            n72 = case shown="\"UserManagement\"" w179 {
              tunnel: [_ "User Menu: Login" "User Menu: Logout" "User Menu: UserManagement" "User Menu: StationOptions" w189 w190 w191 w192 "TestOperation: SelectProductModel" "TestOperation: LunchTest" "User Menu: About" w196 w197 w198] -> w180
              frame "Idle", Default {
              }
              frame "Login" {
              }
              frame "Logout" {
              }
              frame "UserManagement" {
              }
              frame "StationOptions" {
              }
              frame "StepLimitSetting" {
                w189 = "User Menu: StepLimitSetting"  # User Menu: StepLimitSetting
              }
              frame "InstrumentCommunicationSetting" {
                w190 = "User Menu: InstrumentCommunicationSetting"  # User Menu: InstrumentCommunicationSetting
              }
              frame "LogView" {
                w191 = "User Menu: LogView"  # User Menu: LogView
              }
              frame "DataAnalysis" {
                w192 = "User Menu: DataAnalysis"  # User Menu: DataAnalysis
              }
              frame "ChangeProductModel" {
              }
              frame "LunchTest" {
              }
              frame "About" {
              }
              frame "Terminate" {
                w196 = "User Menu: Terminate"  # User Menu: Terminate
              }
              frame "DebugUI" {
                w197 = "User Menu: DebugUI"  # User Menu: DebugUI
              }
              frame "TestParameterEdit" {
                w198 = "User Menu: TestParameterEdit"  # User Menu: TestParameterEdit
              }
            }
            n73 = call <vilib>:"Add State(s) to Queue__JKI_lib_State_Machine.vi"("State(s) in (\"\")"=w184, "State(s) at Back (\"\")"=w180) -> ("States Out"=w183:string)  [unwired: 13 in]
          }
        }
      }
      frame "---------- Core ----------" {
        n74 = call <vilib>:"Add State(s) to Queue__JKI_lib_State_Machine.vi"("State(s) in (\"\")"=w203) -> ("States Out"=w202:string)  [unwired: 14 in]
      }
      frame Default {
        w214 = 42 items=["No error", "Argument error", "Memory is full", "Out of zone", "End of file", "File already open", "Generic file I/O error", "File not found", "File permission error", "Disk is full", "Duplicate path", "Too many files open", "System feature not enabled", "Resource file not found", "Cannot add resource", "Resource not found", "Image not found", "Image memory error", "Pen does not exist", "Config type invalid", "Config token not found", "Config parse error", "Config memory error", "Bad external code format", "Bad external code offset", "External code not present", "Null window", "Destroy window error", "Null menu", "Print aborted", "Bad print record", "Print driver error", "Windows error during printing", "Memory error during printing", "Print dialog error", "Generic print error", "Invalid device refnum", "Device not found", "Device parameter error", "Device unit error", "Cannot open device", "Device call aborted", "Generic error", "Cancelled by user", "Object ID too low", "Object ID too high", "Object not in heap", "Unknown heap", "Unknown object (invalid DefProc)", "Unknown object (DefProc not in table)", "Message out of range", "Invalid (null) method", "Unknown message", "Manager call not supported", "Bad address", "Network operation in progress", "Network operation timed out", "Connection is busy", "Network attribute not supported", "Network error", "Address in use", "System out of memory", "Connection aborted", "Connection refused", "Not connected", "Already connected", "Connection closed", "Initialization error (interapplication manager)", "Bad occurrence", "Wait on unbound occurrence handler", "Occurrence queue overflow", "Datalog type conflict", "Unused", "Unrecognized type (interapplication manager)", "Memory corrupt", "Failed to make temporary DLL", "Old CIN version", "Drag socket not found", "Failed to load drop-object", "Failed to register OLE object", "Failed to release OLE object", "Format specifier type mismatch", "Unknown format specifier", "Too few format specifiers", "Too many format specifiers", "Scan failed", "Newer CIN version", "Error converting to variant", "Runtime menu error", "Password tampered", "Variant attribute not found", "Incompatible variant data type", "Event data is not available", "Event Store is not present", "Occurrence is not found", "Event Queue is not created", "Event info is not available", "Refnum passed is NULL", "Error retrieving Class GUID", "Error retrieving CoClass GUID", "Error retrieving TypeLib GUID.", "Bad built application magic bytes.", "Specific driver is different from the specific driver associated with the Logical Name.", "There is no session opened to the class driver.", "Max Error", "MAX - Error with config objects", "MAX - Error loading configuration", "MAX - Group not supported"]
        # "Current State"
        # "Handle mistyped state name (developer tool)"
        n75 = Format Into String(format string="Software Exception: Unhandled State \"%s\"." ("message"), error in=w210, w205) -> (resulting string=w213:string, error out=w212:errorcluster)  [unwired: 1 in]
        n76 = call <vilib>:"Error Cluster From Error Code.vi"("show call chain? (False)"=TRUE, "error in (no error)"=w212, "error message (\"\")"=w213, "error code (0)"=w214) -> ("error out"=w211:errorcluster)  [unwired: 5 in]
        n77 = call <vilib>:"Add State(s) to Queue__JKI_lib_State_Machine.vi"("State(s) in (\"\")"=w209) -> ("States Out"=w208:string)  [unwired: 14 in]
      }
      frame "Initialize Core Data" {
        # "Do not delete, rename, or modify this frame.\n(this is used to determine panel behavior on exit)"
        # "originally closed?"
        # "exe?"
        # "If panel starts closed or is an EXE, then close it when we exit"
        n78 = property class="VI"() -> ("FP.State"=w219:T10)  [unwired: 2 in, 2 out]
        n79 = property class="App"() -> ("App.Kind"=w225:T11)  [unwired: 2 in, 2 out]
        n80 = control-ref of="Current VI Reference"() -> (w220:refnum<vi>)
        n81 = Equal?(x=w219, y=T10."Closed" ("Front Panel Window:State")) -> (x = y?=w217:bool)
        n82 = Equal?(x=w225, y=T11."Run Time System" ("Application:Kind")) -> (x = y?=w223:bool)
        n83 = Or(x=w217, y=w223) -> (x .or. y?=w221:bool)
        n84 = Bundle By Name(cluster=w222, "Core.Current VI Reference"=w220, "Core.Close Panel on Exit?"=w221) -> (w227:T13)
        n85 = call <vilib>:"Add State(s) to Queue__JKI_lib_State_Machine.vi"("State(s) in (\"\")"=w229) -> ("States Out"=w228:string)  [unwired: 14 in]
      }
      frame "Error Handler" {
        # "Unhandled Error -- Display it"
        # "Handle any errors here.\nYou can also output any states to clean-up after errors occur"
        # "Clear error"
        n86 = call <vilib>:"General Error Handler.vi"("error in (no error)"=w232) -> ()  [unwired: 10 in, 5 out]
        n87 = call <vilib>:"Add State(s) to Queue__JKI_lib_State_Machine.vi"("State(s) in Front (\"\")"="/* Post Error States", "State(s) in (\"\")"=w236) -> ("States Out"=w235:string)  [unwired: 13 in]
      }
      frame "Exit" {
        # "Do not put any code in this frame.\n(No errors that occur here will be handled.)"
        n88 = call "Send Stop Test Engine Actor.vi"("Message Enqueuer"=w238) -> ("Message Enqueuer out"=w237:refnum<class "Message Enqueuer.lvclass">)  [unwired: 9 in, 1 out]
        n89 = Build Array(w247, w246, w245, w244, w243, w242, w241, w240, w237) -> (w239:refnum<class "Message Enqueuer.lvclass">[])
        n90 = for {
          tunnel: w239 -> [w254] mode=indexing
          n91 = call <vilib>:"Send Normal Stop.vi"("Message Enqueuer"=w254) -> ()  [unwired: 10 in, 1 out]
        }
        n92 = call <vilib>:"Add State(s) to Queue__JKI_lib_State_Machine.vi"("State(s) in (\"\")"=w253) -> ("States Out"=w252:string)  [unwired: 14 in]
      }
      frame "---------- Data ----------" {
        # "Do not put any code in this frame.\n(It is a separator no-op. You can make a copy of this frame to create a new Data frame)"
        n93 = call <vilib>:"Add State(s) to Queue__JKI_lib_State_Machine.vi"("State(s) in (\"\")"=w259) -> ("States Out"=w258:string)  [unwired: 14 in]
      }
      frame "Data: Initialize" {
        w263 = T3 {"Report Path"=path "", "Report  Format"=enum."CSV", "Disabled State"=FALSE, "Customer name"=""}  # Local Report
        w264 = T2 {"Connection String Expression"="", "User ID"="", "Password"=""}  # DataBase
        w266 = T14 {"Current VI Reference"=refnum, "Close Panel on Exit?"=FALSE}  # Core
        # "Initialize the shift-register data, here.\n(data names are defined by what you wire into the bundle function)"
        n94 = Bundle("Core"=w266, "DataBase"=w264, "Local Report"=w263, "Localization"=T4 {"Language"=enum."English"}, "Preferences"=T5 {"Station ID"="", "IP Address"="", "Password"=""}, "User Manager"=T6 {"Current User Manager File"="", "Login on start"=FALSE}) -> (w268:T13)  [unwired: 1 in]
        n95 = call <vilib>:"Add State(s) to Queue__JKI_lib_State_Machine.vi"("State(s) in (\"\")"=w270) -> ("States Out"=w269:string)  [unwired: 14 in]
      }
      frame "Data: Cleanup" {
        # "Cleanup any data and references, here.\n(this is called automatically, by the Macro: Exit)"
        n96 = Unbundle By Name(w272) -> ("Core.Current VI Reference"=w275:refnum<vi>)
        n97 = Close Reference(reference=w275, error in (no error)=w274) -> (error out=w273:errorcluster)
        n98 = call <vilib>:"Add State(s) to Queue__JKI_lib_State_Machine.vi"("State(s) in (\"\")"=w277) -> ("States Out"=w276:string)  [unwired: 14 in]
      }
      frame "---------- Events ----------" {
        # "Do not put any code in this frame.\n(It is a separator no-op. You can make a copy of this frame to create a new UI frame)"
        n99 = call <vilib>:"Add State(s) to Queue__JKI_lib_State_Machine.vi"("State(s) in (\"\")"=w282) -> ("States Out"=w281:string)  [unwired: 14 in]
      }
      frame "Events: Register" {
        n100 = Build Array(w294, w289, w288, w287, w286, w285, w284, w283) -> (w293:refnum<class "Message Enqueuer.lvclass">[])
        n101 = call "RegisterEvents.vi"("Error In"=w291, "Root Actor's Enqueuer"=w292, "Nested Actor's EnqueuerArray"=w293) -> ("Error Out"=w290:errorcluster)  [unwired: 8 in]
        n102 = call <vilib>:"Add State(s) to Queue__JKI_lib_State_Machine.vi"("State(s) in (\"\")"=w298) -> ("States Out"=w297:string)  [unwired: 14 in]
      }
      frame "Events: Unregister" {
        # "Do not put any code in this frame.\n(It is a separator no-op. You can make a copy of this frame to create a new UI frame)"
        n103 = Build Array(w308, w307, w306, w305, w304, w303, w302, w301) -> (w300:refnum<class "Message Enqueuer.lvclass">[])
        n104 = call "UnregisterEvents.vi"("Root Actor's Enqueuer"=w299, "Nested Actor's EnqueuerArray"=w300) -> ()  [unwired: 9 in, 1 out]
        n105 = Unregister For Events(event registration refnum=w311, error in=w310) -> (error out=w309:errorcluster)
        n106 = call <vilib>:"Add State(s) to Queue__JKI_lib_State_Machine.vi"("State(s) in (\"\")"=w314) -> ("States Out"=w313:string)  [unwired: 14 in]
      }
      frame "---------- UI ----------" {
        # "Do not put any code in this frame.\n(It is a separator no-op. You can make a copy of this frame to create a new UI frame)"
        n107 = call <vilib>:"Add State(s) to Queue__JKI_lib_State_Machine.vi"("State(s) in (\"\")"=w319) -> ("States Out"=w318:string)  [unwired: 14 in]
      }
      frame "UI: Initialize" {
        # "Initialize the User Interface, here.\n(this is called automatically, by the Macro: Init)"
        n108 = call "Send UI Initialize.vi"("Message Enqueuer"=w321) -> ()  [unwired: 9 in, 2 out]
        n109 = call <vilib>:"Add State(s) to Queue__JKI_lib_State_Machine.vi"("State(s) in (\"\")"=w325) -> ("States Out"=w324:string)  [unwired: 14 in]
      }
      frame "UI: Cursor Set" {
        # "Argument"
        # "Set and Unset Cursor Busy.\n(Usage: \"UI: Cursor Set >> Busy|Idle\")"
        n110 = case shown="\"Idle\", Default" w327 {
          tunnel: w329 -> [w334 w336]
          tunnel: [w333 w335] -> w328
          frame "Idle", Default {
            n111 = call <vilib>:"Unset Busy.vi"("error in (no error)"=w334) -> ("error out"=w333:errorcluster)  [unwired: 10 in]
          }
          frame "Busy" {
            n112 = call <vilib>:"Set Busy.vi"("error in (no error)"=w336) -> ("error out"=w335:errorcluster)  [unwired: 9 in, 1 out]
          }
        }
        n113 = call <vilib>:"Add State(s) to Queue__JKI_lib_State_Machine.vi"("State(s) in (\"\")"=w332) -> ("States Out"=w331:string)  [unwired: 14 in]
      }
      frame "UI: Localization" {
        # "Do not put any code in this frame.\n(It is a separator no-op. You can make a copy of this frame to create a new UI frame)"
        n114 = call <vilib>:"Add State(s) to Queue__JKI_lib_State_Machine.vi"("State(s) in (\"\")"=w341) -> ("States Out"=w340:string)  [unwired: 14 in]
      }
      frame "UI: Front Panel State" {
        # "Argument"
        # "Set Front Panel Open or Closed\n(Usage: \"UI: Front Panel State >> Open|Close\")"
        n115 = Unbundle By Name(w346) -> ("Core.Current VI Reference"=w343:refnum<vi>)
        n116 = case shown="\"Close\", \"Closed\"" w345 {
          tunnel: w347 -> [w355 w370 w381 w394 w407]
          tunnel: [w357 w371 w383 w396 w409] -> w342
          tunnel: w343 -> [w356 w368 w382 w395 w408]
          frame "Open", "Standard", Default {
            w350 = T10."Standard" ("State")
            n117 = property class="VI"(reference=w356, error in=w355) -> (reference out=w353:refnum<vi>, error out=w354:errorcluster, "FP.State"=w352:T10)
            n118 = Not Equal?(x=w352, y=w350) -> (x != y?=w351:bool)
            n119 = case shown="True" w351 {
              tunnel: [w361 w363] -> w357
              tunnel: w354 -> [w360 w363]
              tunnel: w353 -> [w359 _]
              tunnel: w350 -> [w358 _]
              frame True {
                n120 = invoke class="VI" method="FP.Open"(reference=w359, error in=w360, "Activate"=TRUE, "State"=w358) -> (error out=w361:errorcluster)  [unwired: 1 in, 4 out]
              }
              frame False {
              }
            }
          }
          frame "Close", "Closed" {
            n121 = property class="VI"(reference=w368, error in=w370) -> (reference out=w367:refnum<vi>, error out=w369:errorcluster, "FP.State"=w365:T10)
            n122 = Not Equal?(x=w365, y=T10."Closed" ("Front Panel Window:State")) -> (x != y?=w364:bool)
            n123 = case shown="True" w364 {
              tunnel: [w372 w375] -> w371
              tunnel: w369 -> [w372 w374]
              tunnel: w367 -> [_ w373]
              frame False {
              }
              frame True {
                n124 = invoke class="VI" method="FP.Close"(reference=w373, error in=w374) -> (error out=w375:errorcluster)  [unwired: 1 in, 2 out]
              }
            }
          }
          frame "Hidden", "Hide" {
            w376 = T10."Hidden" ("State")
            n125 = property class="VI"(reference=w382, error in=w381) -> (reference out=w379:refnum<vi>, error out=w380:errorcluster, "FP.State"=w378:T10)
            n126 = Not Equal?(x=w378, y=w376) -> (x != y?=w377:bool)
            n127 = case shown="True" w377 {
              tunnel: [w387 w388] -> w383
              tunnel: w380 -> [w386 w388]
              tunnel: w379 -> [w385 _]
              tunnel: w376 -> [w384 _]
              frame True {
                n128 = invoke class="VI" method="FP.Open"(reference=w385, error in=w386, "State"=w384) -> (error out=w387:errorcluster)  [unwired: 2 in, 4 out]
              }
              frame False {
              }
            }
          }
          frame "Minimize", "Minimized" {
            w389 = T10."Minimized" ("State")
            n129 = property class="VI"(reference=w395, error in=w394) -> (reference out=w392:refnum<vi>, error out=w393:errorcluster, "FP.State"=w391:T10)
            n130 = Not Equal?(x=w391, y=w389) -> (x != y?=w390:bool)
            n131 = case shown="True" w390 {
              tunnel: [w400 w401] -> w396
              tunnel: w393 -> [w399 w401]
              tunnel: w392 -> [w398 _]
              tunnel: w389 -> [w397 _]
              frame True {
                n132 = invoke class="VI" method="FP.Open"(reference=w398, error in=w399, "State"=w397) -> (error out=w400:errorcluster)  [unwired: 2 in, 4 out]
              }
              frame False {
              }
            }
          }
          frame "Maximize", "Maximized" {
            w402 = T10."Maximized" ("State")
            n133 = property class="VI"(reference=w408, error in=w407) -> (reference out=w405:refnum<vi>, error out=w406:errorcluster, "FP.State"=w404:T10)
            n134 = Not Equal?(x=w404, y=w402) -> (x != y?=w403:bool)
            n135 = case shown="True" w403 {
              tunnel: [w413 w414] -> w409
              tunnel: w406 -> [w412 w414]
              tunnel: w405 -> [w411 _]
              tunnel: w402 -> [w410 _]
              frame True {
                n136 = invoke class="VI" method="FP.Open"(reference=w411, error in=w412, "State"=w410) -> (error out=w413:errorcluster)  [unwired: 2 in, 4 out]
              }
              frame False {
              }
            }
          }
        }
        n137 = call <vilib>:"Add State(s) to Queue__JKI_lib_State_Machine.vi"("State(s) in (\"\")"=w349) -> ("States Out"=w348:string)  [unwired: 14 in]
      }
      frame "---------- Macro ----------" {
        # "Do not put any code in this frame.\n(It is a separator no-op. You can make a copy of this frame to create a new Macro frame)"
        n138 = call <vilib>:"Add State(s) to Queue__JKI_lib_State_Machine.vi"("State(s) in (\"\")"=w419) -> ("States Out"=w418:string)  [unwired: 14 in]
      }
      frame "Macro: Initialize" {
        # "Initialization Macro\n(This is called once, when the VI starts)"
        n139 = call <vilib>:"Add State(s) to Queue__JKI_lib_State_Machine.vi"("State(s) in Front (\"\")"="Data: Initialize\nInitialize Core Data\nEvents: Register\nUI: Initialize\nUser Menu: Logout\nUI: Front Panel State >> Maximize", "State(s) in (\"\")"=w425) -> ("States Out"=w424:string)  [unwired: 13 in]
      }
      frame "Macro: Exit" {
        # "Exit Macro\n(This is called once, when the VI exits)"
        n140 = Unbundle By Name(w433) -> ("Core.Close Panel on Exit?"=w432:bool)
        n141 = Select(t="UI: Front Panel State >> Close", s=w432, f="") -> (s? t:f=w429:string)
        n142 = call <vilib>:"Add State(s) to Queue__JKI_lib_State_Machine.vi"("State(s) in (\"\")"=w429, "State(s) at Back (\"\")"="Data: Cleanup\nEvents: Unregister\nExit") -> ("States Out"=w427:string)  [unwired: 13 in]
        n143 = call <vilib>:"Add State(s) to Queue__JKI_lib_State_Machine.vi"("State(s) in Front (\"\")"=w427, "State(s) in (\"\")"=w436) -> ("States Out"=w435:string)  [unwired: 13 in]
      }
      frame "---------- User Menu ----------" {
        # "Template Separator\n(You can make a copy of, or modify, this frame)"
        n144 = call <vilib>:"Add State(s) to Queue__JKI_lib_State_Machine.vi"("State(s) in (\"\")"=w441) -> ("States Out"=w440:string)  [unwired: 14 in]
      }
      frame "User Menu: Login" {
        # "Your code here.\n(You can make a copy of, or modify, this frame)"
        n145 = call "Send Login.vi"("Message Enqueuer"=w443) -> ()  [unwired: 9 in, 2 out]
        n146 = call <vilib>:"Add State(s) to Queue__JKI_lib_State_Machine.vi"("State(s) in (\"\")"=w447) -> ("States Out"=w446:string)  [unwired: 14 in]
      }
      frame "User Menu: Logout" {
        # "Your code here.\n(You can make a copy of, or modify, this frame)"
        n147 = call "Send Logout.vi"("Message Enqueuer"=w448) -> ()  [unwired: 9 in, 2 out]
        n148 = call <vilib>:"Add State(s) to Queue__JKI_lib_State_Machine.vi"("State(s) in (\"\")"=w453) -> ("States Out"=w452:string)  [unwired: 14 in]
      }
      frame "User Menu: UserManagement" {
        # "Your code here.\n(You can make a copy of, or modify, this frame)"
        n149 = call "Send ActorCoreMassageEvent.vi"("ActorCoreEventMassage"="OpenFrontPanel", "Message Enqueuer"=w455) -> ()  [unwired: 8 in, 2 out]
        n150 = call <vilib>:"Add State(s) to Queue__JKI_lib_State_Machine.vi"("State(s) in (\"\")"=w460) -> ("States Out"=w459:string)  [unwired: 14 in]
      }
      frame "User Menu: StationOptions" {
        # "Your code here.\n(You can make a copy of, or modify, this frame)"
        n151 = call "Send ActorCoreEvent.vi"("ActorCoreMessage"="OpenFrontPanel" ("ActorCoreEventMassage"), "Message Enqueuer"=w462) -> ()  [unwired: 8 in, 2 out]
        n152 = call <vilib>:"Add State(s) to Queue__JKI_lib_State_Machine.vi"("State(s) in (\"\")"=w467) -> ("States Out"=w466:string)  [unwired: 14 in]
      }
      frame "User Menu: StepLimitSetting" {
        # "Your code here.\n(You can make a copy of, or modify, this frame)"
        n153 = call "Send ActorCoreEvent.vi"("ActorCoreMessage"="OpenFrontPanel" ("ActorCoreEventMassage"), "Message Enqueuer"=w468) -> ()  [unwired: 8 in, 2 out]
        n154 = call <vilib>:"Add State(s) to Queue__JKI_lib_State_Machine.vi"("State(s) in (\"\")"=w474) -> ("States Out"=w473:string)  [unwired: 14 in]
      }
      frame "User Menu: InstrumentCommunicationSetting" {
        # "Your code here.\n(You can make a copy of, or modify, this frame)"
        n155 = call "Send ActorCoreEvent.vi"("ActorCoreMessage"="OpenFrontPanel" ("ActorCoreEventMassage"), "Message Enqueuer"=w475) -> ()  [unwired: 8 in, 2 out]
        n156 = call <vilib>:"Add State(s) to Queue__JKI_lib_State_Machine.vi"("State(s) in (\"\")"=w481) -> ("States Out"=w480:string)  [unwired: 14 in]
      }
      frame "User Menu: LogView" {
        # "Your code here.\n(You can make a copy of, or modify, this frame)"
        n157 = call "Send ActorCoreEvent.vi"("ActorCoreMessage"="OpenFrontPanel" ("ActorCoreEventMassage"), "Message Enqueuer"=w483) -> ()  [unwired: 8 in, 2 out]
        n158 = call <vilib>:"Add State(s) to Queue__JKI_lib_State_Machine.vi"("State(s) in (\"\")"=w488) -> ("States Out"=w487:string)  [unwired: 14 in]
      }
      frame "User Menu: DataAnalysis" {
        # "Your code here.\n(You can make a copy of, or modify, this frame)"
        n159 = call "Send ActorCoreEvent.vi"("Message"="OpenFrontPanel" ("ActorCoreEventMassage"), "Message Enqueuer"=w490) -> ()  [unwired: 8 in, 2 out]
        n160 = call <vilib>:"Add State(s) to Queue__JKI_lib_State_Machine.vi"("State(s) in (\"\")"=w495) -> ("States Out"=w494:string)  [unwired: 14 in]
      }
      frame "User Menu: About" {
        # "Your code here.\n(You can make a copy of, or modify, this frame)"
        n161 = One Button Dialog(message="Software version: 1.0.0.9\n----------------------------\nXXW Engineer\nPhone: 17625347372\nE-mail: x.xw1991@163.com") -> ()  [unwired: 1 in, 1 out]
        n162 = call <vilib>:"Add State(s) to Queue__JKI_lib_State_Machine.vi"("State(s) in (\"\")"=w501) -> ("States Out"=w500:string)  [unwired: 14 in]
      }
      frame "User Menu: Terminate" {
        # "Your code here.\n(You can make a copy of, or modify, this frame)"
        n163 = call "Send Terminate Test.vi"("Message Enqueuer"=w502) -> ()  [unwired: 9 in, 2 out]
        n164 = call <vilib>:"Add State(s) to Queue__JKI_lib_State_Machine.vi"("State(s) in (\"\")"=w507) -> ("States Out"=w506:string)  [unwired: 14 in]
      }
      frame "User Menu: DebugUI" {
        # "Your code here.\n(You can make a copy of, or modify, this frame)"
        n165 = call <vilib>:"Application Directory.vi"() -> ("Application Directory"=w516:path)
        n166 = Build Path(base path=w516, name or relative path="DebugUI") -> (appended path=w514:path)
        n167 = Build Path(base path=w514, name or relative path="DebugUI.exe") -> (appended path=w510:path)
        n168 = call <vilib>:"Check if File or Folder Exists.vi"("path"=w510) -> ("file or folder exists?"=w508:bool, "dup path"=w509:path)  [unwired: 8 in, 1 out]
        n169 = Path To String(path=w509) -> (string=w512:string)
        n170 = case shown="False" w508 {
          tunnel: w517 -> [w523 w527]
          tunnel: w512 -> [_ w525]
          tunnel: [w523 w524] -> w511
          frame False {
            n171 = One Button Dialog(message="DebugUI not found !") -> ()  [unwired: 1 in, 1 out]
          }
          frame True {
            n172 = call <vilib>:"System Exec.vi"("error in (no error)"=w527, "command line"=w525) -> ("error out"=w526:errorcluster)  [unwired: 6 in, 3 out]
            n173 = call <vilib>:"Clear Errors.vi"("error in (no error)"=w526) -> ("error out"=w524:errorcluster)  [unwired: 5 in, 1 out]
          }
        }
        n174 = call <vilib>:"Add State(s) to Queue__JKI_lib_State_Machine.vi"("State(s) in (\"\")"=w521) -> ("States Out"=w520:string)  [unwired: 14 in]
      }
      frame "User Menu: TestParameterEdit" {
        # "Your code here.\n(You can make a copy of, or modify, this frame)"
        n175 = call <vilib>:"Application Directory.vi"() -> ("Application Directory"=w537:path)
        n176 = Build Path(base path=w537, name or relative path="DebugUI") -> (appended path=w535:path)
        n177 = Build Path(base path=w535, name or relative path="Test Parameter Edit.exe") -> (appended path=w532:path)
        n178 = call <vilib>:"Check if File or Folder Exists.vi"("path"=w532) -> ("file or folder exists?"=w530:bool, "dup path"=w531:path)  [unwired: 8 in, 1 out]
        n179 = Path To String(path=w531) -> (string=w533:string)
        n180 = case shown="True" w530 {
          tunnel: w529 -> [w543 w547]
          tunnel: w533 -> [_ w545]
          tunnel: [w543 w544] -> w528
          frame False {
            n181 = One Button Dialog(message="Test Parameter Edit not found !") -> ()  [unwired: 1 in, 1 out]
          }
          frame True {
            n182 = call <vilib>:"System Exec.vi"("error in (no error)"=w547, "command line"=w545) -> ("error out"=w546:errorcluster)  [unwired: 6 in, 3 out]
            n183 = call <vilib>:"Clear Errors.vi"("error in (no error)"=w546) -> ("error out"=w544:errorcluster)  [unwired: 5 in, 1 out]
          }
        }
        n184 = call <vilib>:"Add State(s) to Queue__JKI_lib_State_Machine.vi"("State(s) in (\"\")"=w541) -> ("States Out"=w540:string)  [unwired: 14 in]
      }
      frame "---------- TestOperation ----------" {
        # "Your code here.\n(You can make a copy of, or modify, this frame)"
        n185 = call <vilib>:"Add State(s) to Queue__JKI_lib_State_Machine.vi"("State(s) in (\"\")"=w552) -> ("States Out"=w551:string)  [unwired: 14 in]
      }
      frame "TestOperation: SelectProductModel" {
        # "Your code here.\n(You can make a copy of, or modify, this frame)"
        n186 = call "Send SelectProductModel.vi"("Message Enqueuer"=w553) -> ()  [unwired: 9 in, 2 out]
        n187 = call <vilib>:"Add State(s) to Queue__JKI_lib_State_Machine.vi"("State(s) in (\"\")"=w558) -> ("States Out"=w557:string)  [unwired: 14 in]
      }
      frame "TestOperation: ReadSerialNumber" {
        # "Your code here.\n(You can make a copy of, or modify, this frame)"
        n188 = call "Send ReadSerialNumber.vi"("Message Enqueuer"=w559) -> ()  [unwired: 9 in, 2 out]
        n189 = call <vilib>:"Add State(s) to Queue__JKI_lib_State_Machine.vi"("State(s) in (\"\")"=w564) -> ("States Out"=w563:string)  [unwired: 14 in]
      }
      frame "TestOperation: LunchTest" {
        # "Your code here.\n(You can make a copy of, or modify, this frame)"
        n190 = Unbundle By Name(w571) -> ("Local Report"=w570:T3)
        n191 = call "Send InitializeReport.vi"("error in (no error)"=w568, "Local Report Parameter"=w570, "Message Enqueuer"=w572) -> ("error out"=w569:errorcluster)  [unwired: 7 in, 1 out]
        n192 = call "Stall Data Flow.vim"("value in"=w569, "milliseconds to wait"=u32 100) -> ("value out"=w566:errorcluster)  [unwired: 1 out]
        n193 = call "Send LunchTest.vi"("error in (no error)"=w566, "Message Enqueuer"=w573) -> ("error out"=w567:errorcluster)  [unwired: 8 in, 1 out]
        n194 = call <vilib>:"Add State(s) to Queue__JKI_lib_State_Machine.vi"("State(s) in (\"\")"=w576) -> ("States Out"=w575:string)  [unwired: 14 in]
      }
      frame "TestOperation: Change Socket" {
        # "Your code here.\n(You can make a copy of, or modify, this frame)"
        n195 = call "Send Change Sub Panel VI.vi"("error in (no error)"=w578, "Message Enqueuer"=w579) -> ("error out"=w577:errorcluster)  [unwired: 8 in, 1 out]
        n196 = call <vilib>:"Add State(s) to Queue__JKI_lib_State_Machine.vi"("State(s) in (\"\")"=w583) -> ("States Out"=w582:string)  [unwired: 14 in]
      }
      frame "TestOperation: PopUp" {
        # "Your code here.\n(You can make a copy of, or modify, this frame)"
        n197 = call "Send PopUp.vi"("error in (no error)"=w585, "Message Enqueuer"=w586) -> ("error out"=w584:errorcluster)  [unwired: 8 in, 1 out]
        n198 = call <vilib>:"Add State(s) to Queue__JKI_lib_State_Machine.vi"("State(s) in (\"\")"=w590) -> ("States Out"=w589:string)  [unwired: 14 in]
      }
      frame "---------- Database ----------" {
        # "Your code here.\n(You can make a copy of, or modify, this frame)"
        n199 = call <vilib>:"Add State(s) to Queue__JKI_lib_State_Machine.vi"("State(s) in (\"\")"=w595) -> ("States Out"=w594:string)  [unwired: 14 in]
      }
      frame "Database: Initialize" {
        n200 = Unbundle By Name(w602) -> ("DataBase.User ID"=w600:string, "DataBase.Connection String Expression"=w599:string, "DataBase.Password"=w598:string)
        n201 = Bundle By Name(cluster=T12 {"User ID"="", "ConnectString"="", "Password"=""} ("ConnectParameter"), "User ID"=w600, "ConnectString"=w599, "Password"=w598) -> (w597:T12)
        n202 = call "Send Initialize.vi"("error in (no error)"=w596, "ConnectParameter"=w597, "Message Enqueuer"=w603) -> ()  [unwired: 7 in, 2 out]
        n203 = call <vilib>:"Add State(s) to Queue__JKI_lib_State_Machine.vi"("State(s) in (\"\")"=w606) -> ("States Out"=w605:string)  [unwired: 14 in]
      }
    }
  }
  n204 = call-parent "Actor Core.vi"("error in"=w6, "Actor in"=w62) -> ("error out"=→"error out":errorcluster, "Actor out"=→"Actor out":refnum<class "Actor.lvclass">)  [unwired: 8 in]
